vi "volume_viewer.vi"() -> ()   [LabVIEW 2024]
uses:
  <vilib>/sklein/WebView2/Webview2 Control/WebView2 Control.xctl
  definitions/local_volume.ctl
  definitions/local_issue.ctl
  definitions/comicvine_issue.generic_credit.ctl
  definitions/comicvine_issue.associated_image.ctl
  definitions/comicvine_issue.person_credit.ctl
  <vilib>/addons/_JKI Toolkits/State Machine/_JKI_lib_State_Machine.llb/Select State(s)_err__jki_lib_state_machine.vi
  <vilib>/addons/_JKI Toolkits/State Machine/_JKI_lib_State_Machine.llb/Periodic Trigger__ogtk__JKI-SM__jki_lib_state_machine.vi
  <userlib>/_OpenG.lib/file/file.llb/Strip Path Extension - String__ogtk.vi
  <userlib>/_OpenG.lib/file/file.llb/openg_file.lvlib
  <vilib>/addons/_JKI.lib/Serialization/JSON/JKI JSON Serialization.lvlib
panel:
  in  "issue detail tab control":enum32{"Details", "Cover", "Lists"}(tab)
  out "Issue ID":i32 caption="Numeric"
  out "Issue Title":string
  out "Cover Date":string
  out "Issue Number":string
  in  "issue description":string(xcontrol)
  in  "issue cover":string(xcontrol)
  out "Characters":string[](array[string])
  out "Teams":string[](array[string])
  out "StoryArcs":string[](array[string])
  out "Creators":string[](array[string])
  out "Concepts":string[](array[string])
  in  "sort volume":bool
  in  "to top":bool
  in  "move down":bool
  in  "move up":bool
  in  "issues":i32(listbox)
  out "Start Year":i32 caption="Numeric"
  out "Number of issues":i32 caption="Numeric"
  out "Sortable Title":string
  out "Title":string
  in  "volume description":string(xcontrol)
  in  "volumes":i32(listbox)
  in  "Folder":i32(listbox)
  in  "Exit":bool
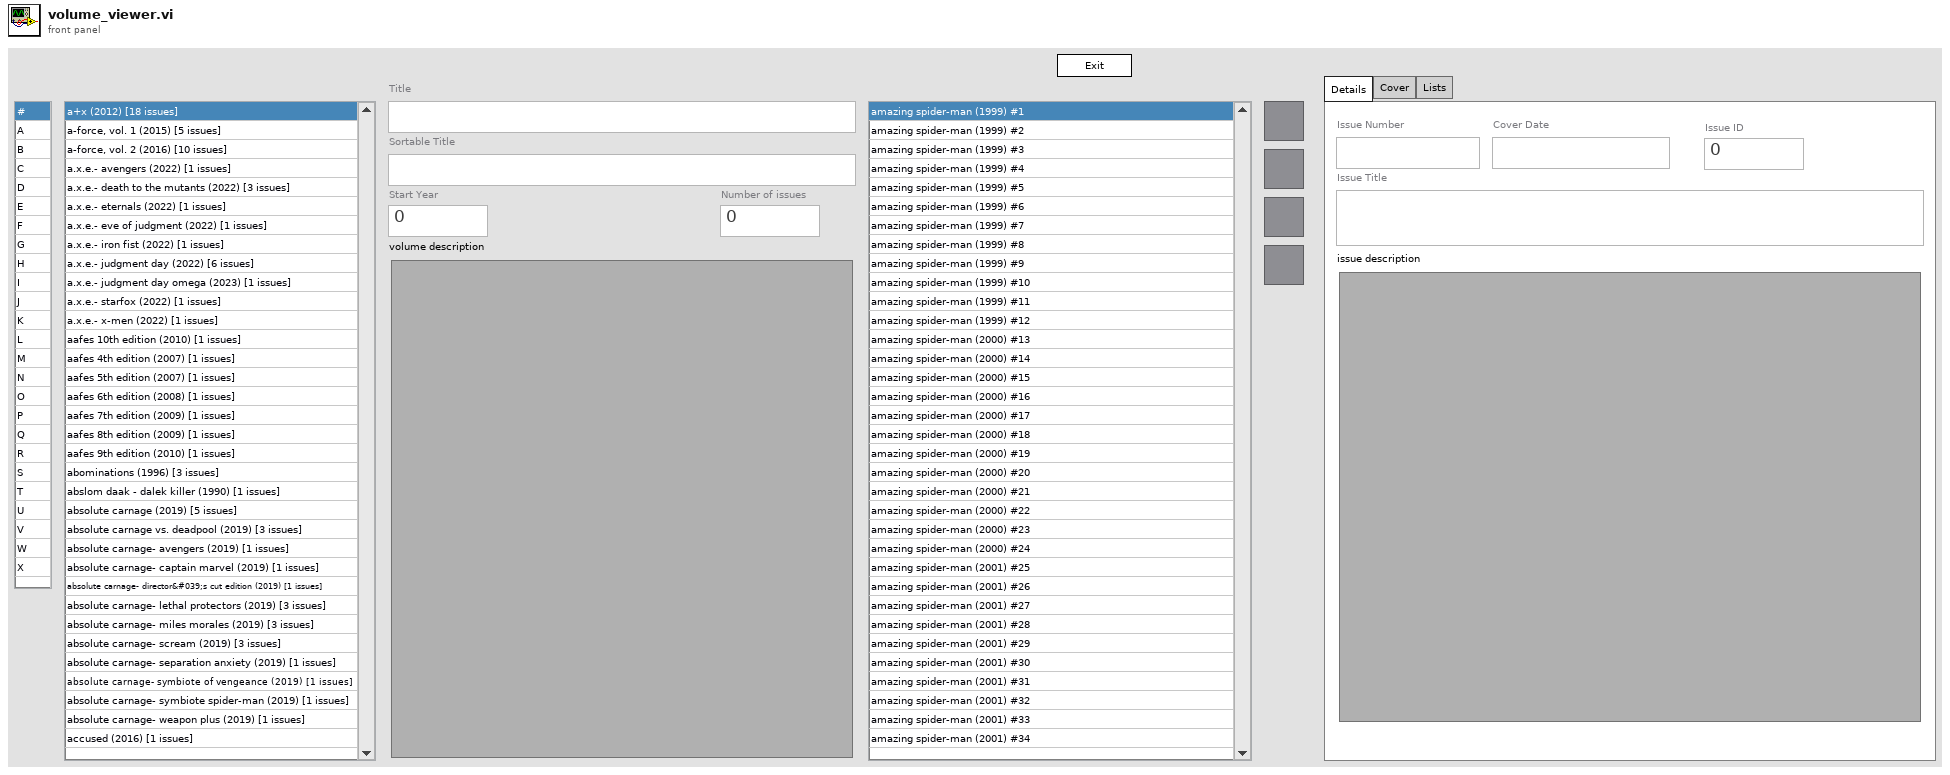
[diagram p1: front panel]
types:
  T1 = enum32{"Invalid", "Standard", "Closed", "Hidden", "Minimized", "Maximized"}
  T2 = enum32{"invalid app kind", "Development System", "Run Time System", "Student Edition", "Embedded LabVIEW", "Evaluation", "Custom"}
  T3 = typedef "local_volume.ctl" = cluster{"id":i32, "name":string, "name_sortable":string, "aliases":string[], "description":string, "url":string, "count_of_issues":i32, "start_year":i32, "publisher_id":i32, "issue_ids":i32[], "date_last_updated":timestamp, "volume":i32, "cv_id":string}
  T4 = typedef "local_issue.ctl" = cluster{"cover_date":timestamp, "id":i32, "cv_id":string, "name":string, "sortable_name":string, "issue_number":string, "deck":string, "description":string, "volume":T5, "store_date":timestamp, "date_last_updated":timestamp, "site_detail_url":string, "cover_url":string, "associated_images":T6[], "characters":T5[], "concepts":T5[], "creators":T7[], "storyArcs":T5[], "teams":T5[]}
  T5 = typedef "comicvine_issue.generic_credit.ctl" = cluster{"id":i32, "name":string}
  T6 = typedef "comicvine_issue.associated_image.ctl" = cluster{"original_url":string, "id":i32}
  T7 = typedef "comicvine_issue.person_credit.ctl" = cluster{"id":i32, "name":string, "role":string}
  T8 = cluster{"Core":cluster{"Current VI Reference":refnum<vi>, "Close Panel on Exit?":bool}, "cv_vols":path[], "vol_filter_map":map{i32, cluster{"name":string, "path":path}[]}, "current_vol_array":cluster{"name":string, "path":path}[], "volume":T3, "issues":T4[], "root paths":cluster{"cv_volumes":path, "cv_issues":path}}
  T9 = cluster{"Current VI Reference":refnum<vi>, "Close Panel on Exit?":bool}
  T10 = typedef "WebView2 Control.xctl/Events.ctl" = cluster{"Navigation Complete Event":refnum<user-event>, "Source Changed Event":refnum<user-event>, "Document Title Changed Event":refnum<user-event>, "Status Bar Text Changed":refnum<user-event>, "Web Message Received":refnum<user-event>, "Window Close Requested":refnum<user-event>, "DOM Loaded":refnum<user-event>, "Navigation Started Event":refnum<user-event>}
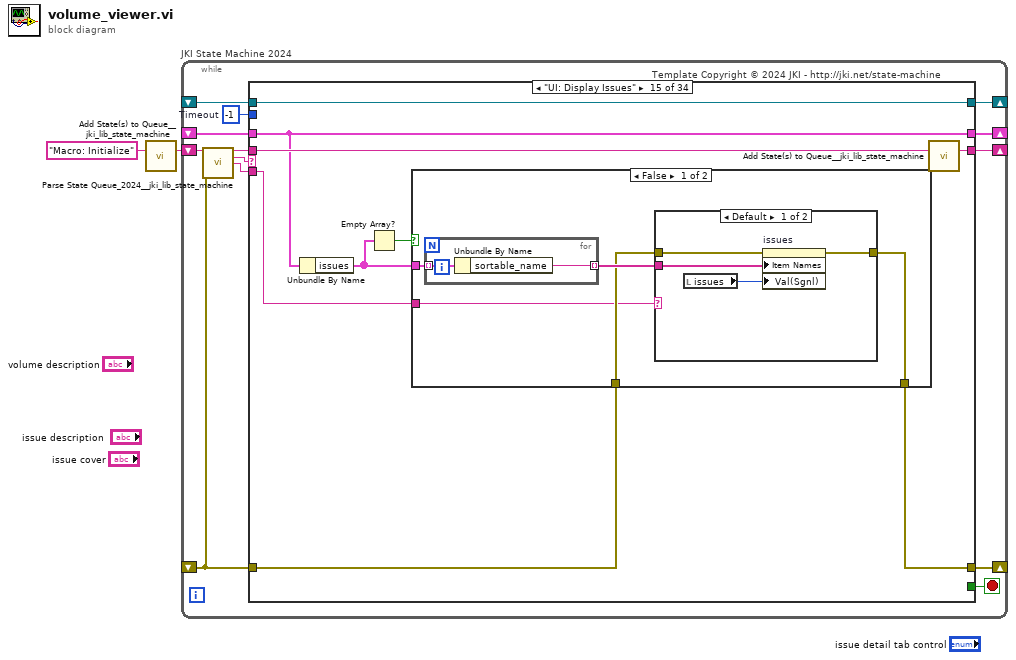
[diagram p0: block diagram]
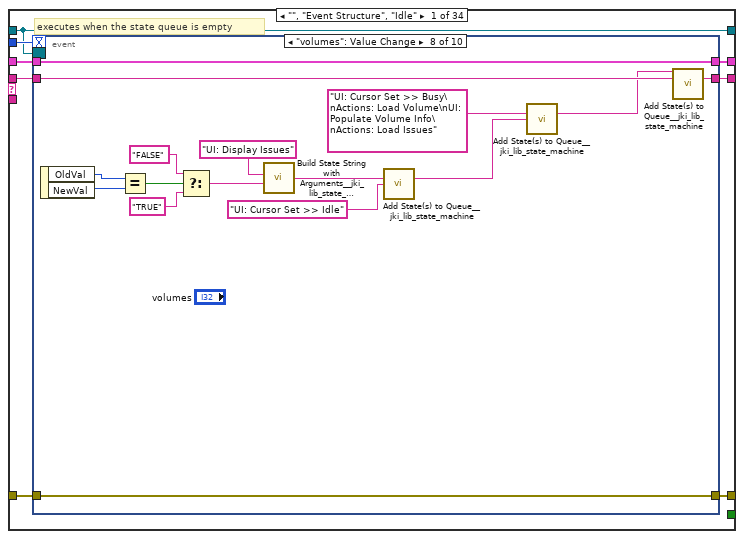
[diagram p2: hidden frame]
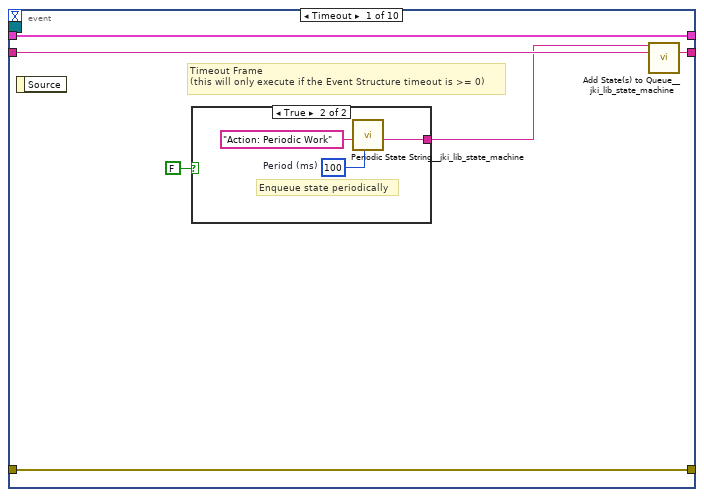
[diagram p3: hidden frame]
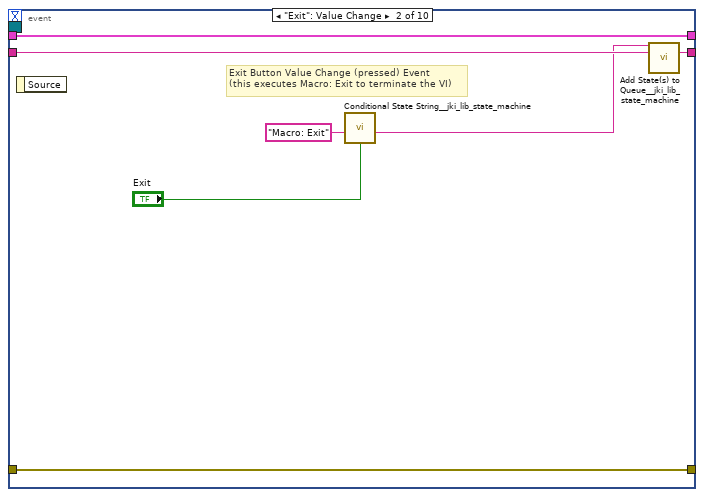
[diagram p5: hidden frame]
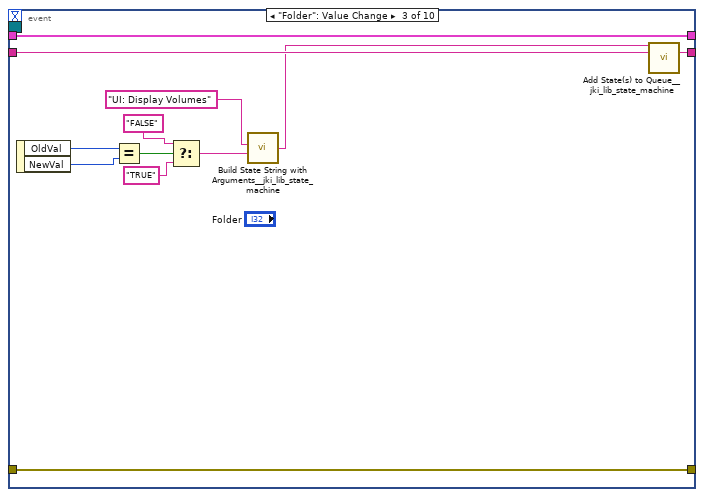
[diagram p6: hidden frame]
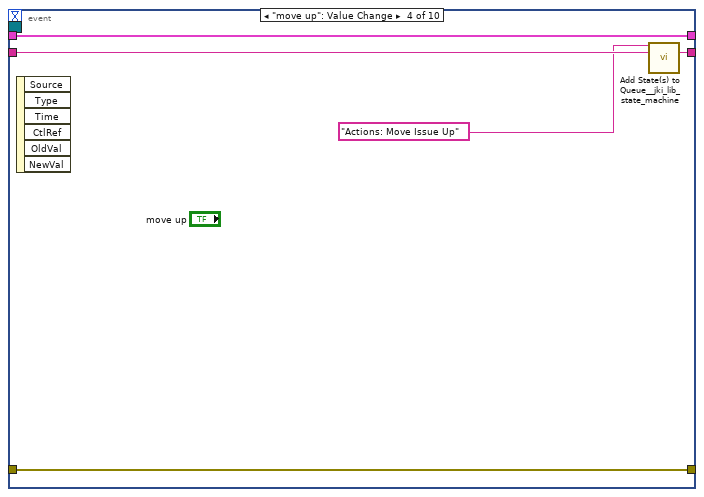
[diagram p7: hidden frame]
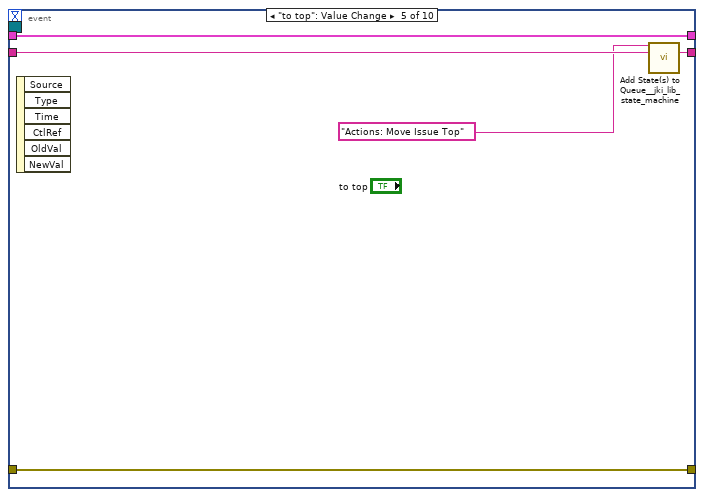
[diagram p8: hidden frame]
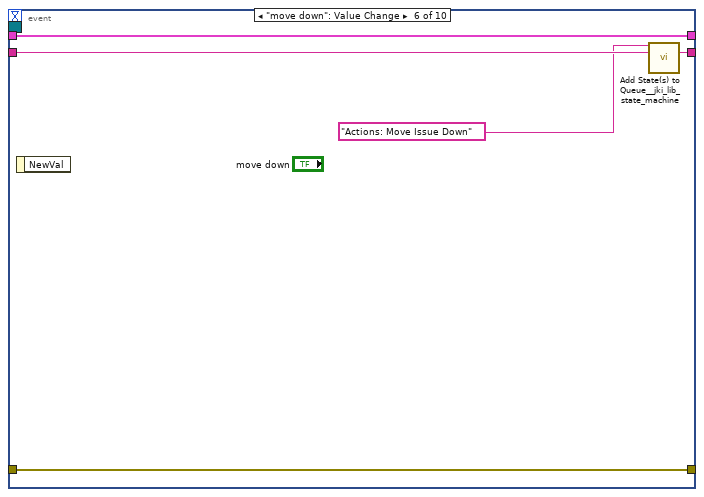
[diagram p9: hidden frame]
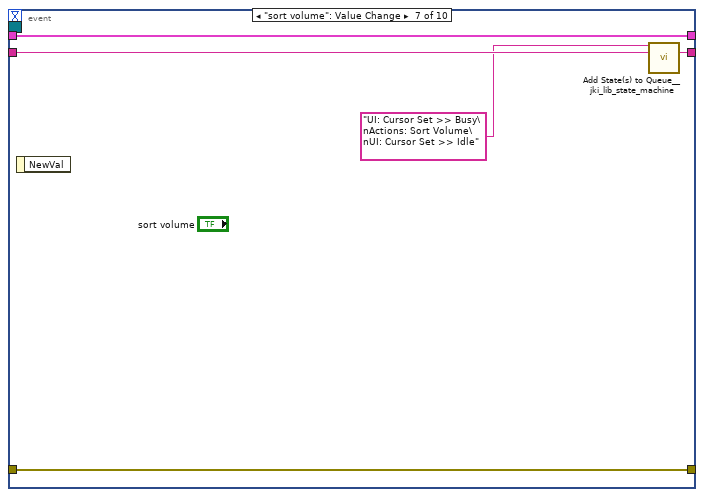
[diagram p10: hidden frame]
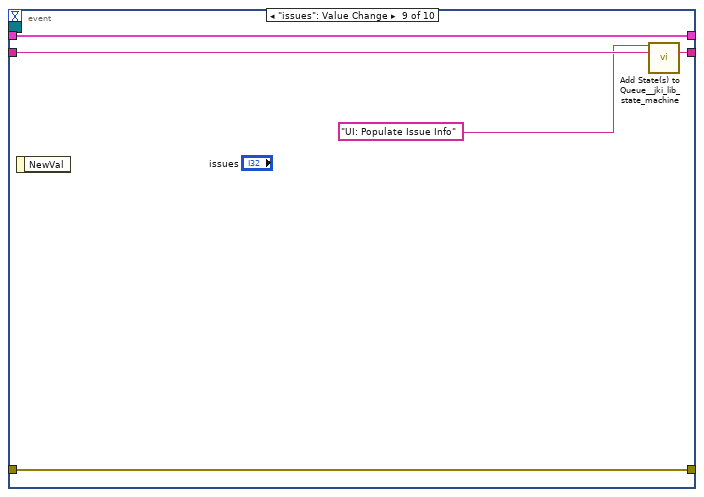
[diagram p11: hidden frame]
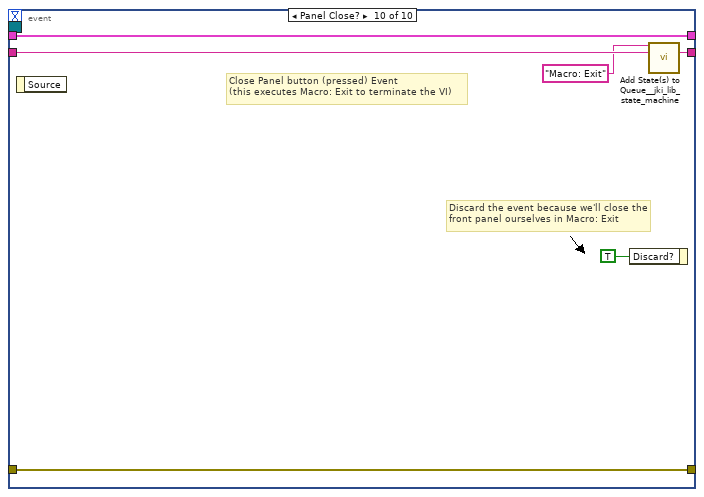
[diagram p12: hidden frame]
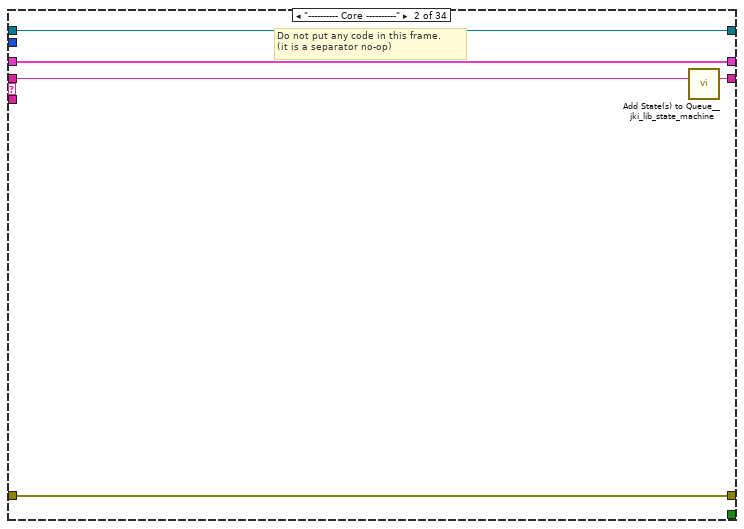
[diagram p13: hidden frame]
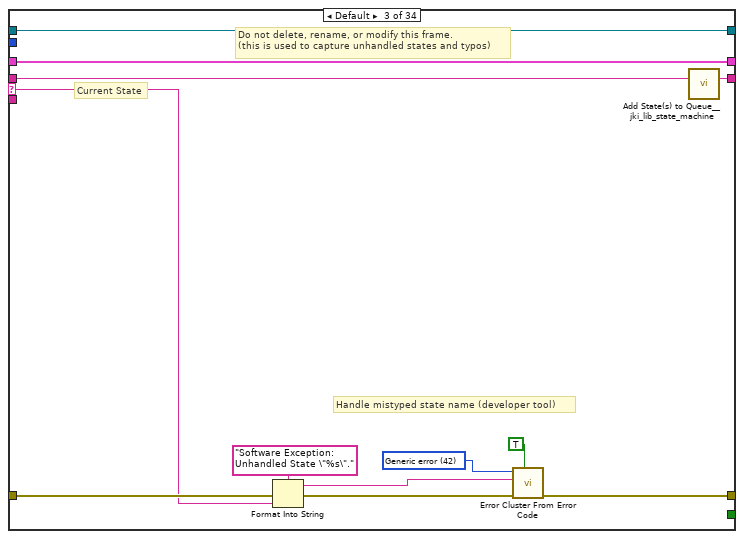
[diagram p14: hidden frame]
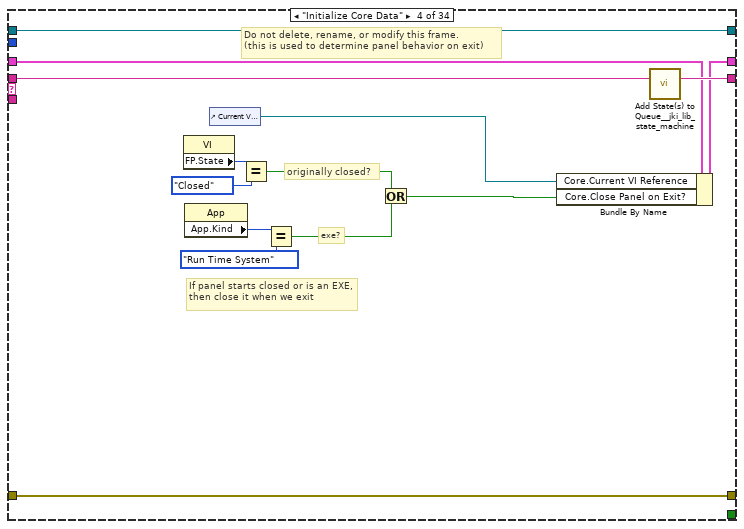
[diagram p15: hidden frame]
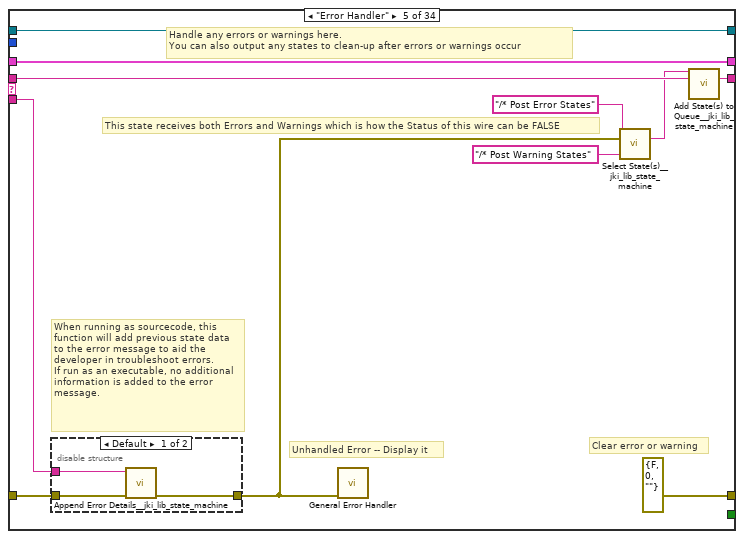
[diagram p16: hidden frame]
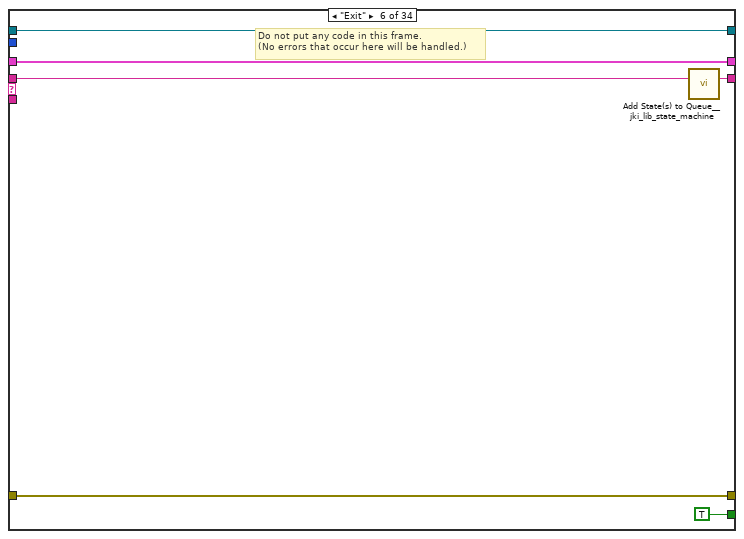
[diagram p18: hidden frame]
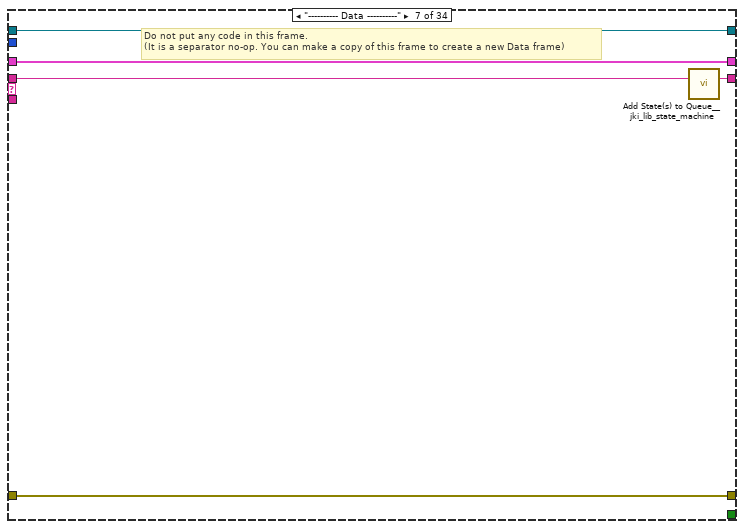
[diagram p19: hidden frame]
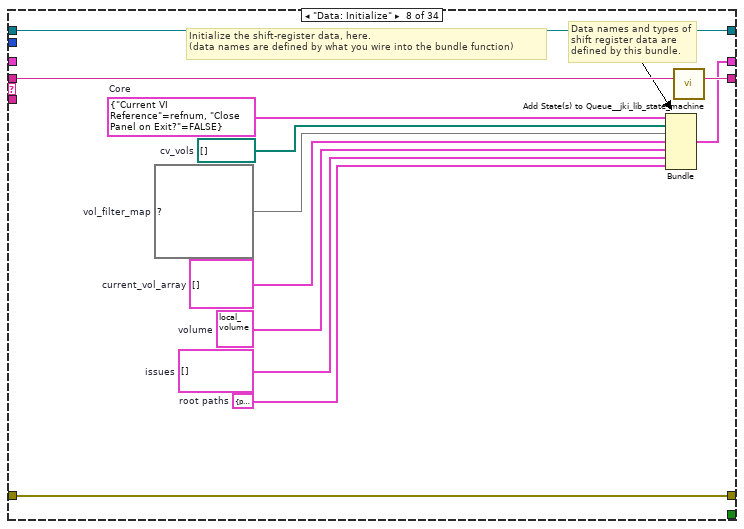
[diagram p20: hidden frame]
diagram:
  n1 = call <vilib>:"Add State(s) to Queue__jki_lib_state_machine.vi"("State(s) in (\"\")"="Macro: Initialize") -> ("States Out"=w2:string)  [unwired: 14 in]
  n2 = while "JKI State Machine 2024" {
    shift-right: [w8] -> _
    shift-left: _ -> [w7]
    shift-right: [w11] -> _
    shift-left: _ -> [w5]
    shift-right: [w10] -> _
    shift-left: w2 -> [w12]
    shift-right: [w4] -> _
    shift-left: _ -> [w3]
    stop <- w9 stop-if-true
    w6 = -1  # Timeout
    # "Template Copyright © 2024 JKI - http://jki.net/state-machine"
    n3 = call <vilib>:"Parse State Queue_2024__jki_lib_state_machine.vi"("State Queue"=w12, "Error In (no error)"=w5) -> ("Remaining States"=w14:string, "Current State"=w15:string, "Arguments"=w13:string)  [unwired: 11 in]
    n4 = case shown="\"UI: Display Issues\"" w15 {
      selector: w15 -> [_ _ w105 _ _ _ _ _ _ _ _ _ _ _ _ _ _ _ _ _ _ _ _ _ _ _ _ _ _ _ _ _ _ _]
      tunnel: w14 -> [w23 w103 w109 w129 w140 w150 w155 w167 w174 w179 w189 w195 w200 w213 w232 w253 w264 w294 w313 w318 w325 w337 w407 w413 w423 w428 w440 w462 w486 w508 w525 w536 w570 w581]
      tunnel: w13 -> [_ _ _ _ w135 _ _ _ _ _ _ _ _ w201 w224 _ _ _ _ _ w320 w331 _ _ _ _ _ _ _ _ _ _ _ _]
      tunnel: w7 -> [w21 w100 w107 w122 w137 w148 w152 _ w169 w176 w187 w193 w197 w209 w227 w250 w259 w291 w311 w316 w323 w333 w404 w410 w421 w425 w436 w459 w483 w505 w511 w530 w562 w576]
      tunnel: [w20 w101 w111 w126 errorcluster {"status"=FALSE, "code"=0, "source"=""} ("error out") w147 w153 w164 w170 w177 w181 w190 w198 w204 w228 w251 w261 w277 w310 w315 w321 w334 w405 w411 w418 w426 w432 w442 w465 w488 w513 w527 w565 w573] -> w11
      tunnel: w5 -> [w17 w101 w110 w126 w136 w147 w153 w164 w171 w177 w183 w191 w198 w205 w229 w251 w262 w280 w310 w315 w322 w335 w405 w411 w418 w426 w437 w449 w473 w495 w519 w531 w564 w572]
      tunnel: [w22 w102 w108 w128 w139 w149 w154 w166 w173 w178 w188 w194 w199 w212 w231 w252 w263 w293 w312 w317 w324 w336 w406 w412 w422 w427 w439 w461 w485 w507 w524 w535 w569 w581] -> w10
      tunnel: [_ _ _ _ _ TRUE _ _ _ _ _ _ _ _ _ _ _ _ _ _ _ _ _ _ _ _ _ _ _ _ _ _ _ _] -> w9
      tunnel: [w19 w100 w107 w127 w137 w148 w152 w165 w169 w176 w187 w193 w197 w208 w227 w250 w259 w291 w311 w316 w323 w333 w404 w410 w421 w425 w436 w459 w483 w505 w510 w528 w566 w574] -> w8
      tunnel: w6 -> [w18 _ _ _ _ _ _ _ _ _ _ _ _ _ _ _ _ _ _ _ _ _ _ _ _ _ _ _ _ _ _ _ _ _]
      tunnel: [w16 w99 w104 w116 w130 w145 w151 w159 w168 w175 w184 w192 w196 w203 w230 w249 w260 w292 w308 w314 w319 w330 w403 w408 w414 w424 w438 w460 w484 w506 w512 w534 w563 w571] -> w4
      tunnel: w3 -> [w16 w99 w104 w116 w130 w145 w151 w159 w168 w175 _ w192 w196 w203 w230 w249 w260 w292 w308 w314 w319 w330 w403 w408 w414 w424 w438 w460 w484 w506 w512 w534 w563 w571]
      frame "", "Event Structure", "Idle" {
        # "executes when the state queue is empty"
        n5 = event shown="[7] \"volumes\": Value Change" {
          selector: w16 -> [_ _ _ _ _ _ _ _ _ _]
          dyn-events: _ -> [_ _ _ _ _ _ _ _ _ _]
          timeout: w18 -> [_ _ _ _ _ _ _ _ _ _]
          tunnel: w23 -> [w29 w39 w51 w56 w61 w66 w71 w87 w92 w98]
          tunnel: [w28 w38 w50 w55 w60 w65 w70 w86 w91 w97] -> w22
          tunnel: w21 -> [w26 w36 w48 w53 w58 w63 w68 w84 w89 w95]
          tunnel: [w27 w37 w49 w54 w59 w64 w69 w85 w90 w96] -> w20
          tunnel: w17 -> [w27 w37 w49 w54 w59 w64 w69 w85 w90 w96]
          tunnel: [w26 w36 w48 w53 w58 w63 w68 w84 w89 w95] -> w19
          event Timeout {
            # "Timeout Frame\n(this will only execute if the Event Structure timeout is >= 0)"
            n6 = event-data() -> ()  [unwired: 1 in, 1 out]
            n7 = case shown="True" FALSE {
              tunnel: [_ w32] -> w25
              frame False {
              }
              frame True {
                w30 = u32 100  # Period (ms)
                # "Enqueue state periodically"
                n8 = call <vilib>:"Periodic State String__jki_lib_state_machine.vi"("Period (ms)"=w30, "State"="Action: Periodic Work") -> ("State Out"=w32:string)  [unwired: 9 in]
              }
            }
            n9 = call <vilib>:"Add State(s) to Queue__jki_lib_state_machine.vi"("State(s) in Front (\"\")"=w25, "State(s) in (\"\")"=w29) -> ("States Out"=w28:string)  [unwired: 13 in]
          }
          event "Exit": Value Change {
            # "Exit Button Value Change (pressed) Event\n(this executes Macro: Exit to terminate the VI)"
            n10 = event-data() -> ()  [unwired: 1 in, 1 out]
            n11 = call <vilib>:"Conditional State String__jki_lib_state_machine.vi"("Do State(s)?"="Exit", "State"="Macro: Exit") -> ("State Out"=w33:string)  [unwired: 7 in]
            n12 = call <vilib>:"Add State(s) to Queue__jki_lib_state_machine.vi"("State(s) in Front (\"\")"=w33, "State(s) in (\"\")"=w39) -> ("States Out"=w38:string)  [unwired: 13 in]
          }
          event "Folder": Value Change {
            n13 = event-data() -> ("OldVal"=w47:i32, "NewVal"=w46:i32)  [unwired: 1 in]
            n14 = Equal?(x=w47, y=w46) -> (x = y?=w45:bool)
            n15 = Select(t="FALSE", s=w45, f="TRUE") -> (s? t:f=w41:string)
            n16 = call <vilib>:"Build State String with Arguments__jki_lib_state_machine.vi"("Arguments (\"\")"=w41, "State"="UI: Display Volumes") -> ("State with Arguments"=w40:string)  [unwired: 4 in]
            n17 = call <vilib>:"Add State(s) to Queue__jki_lib_state_machine.vi"("State(s) in Front (\"\")"=w40, "State(s) in (\"\")"=w51) -> ("States Out"=w50:string)  [unwired: 13 in]
          }
          event "move up": Value Change {
            n18 = event-data() -> ()  [unwired: 1 in, 6 out]
            n19 = call <vilib>:"Add State(s) to Queue__jki_lib_state_machine.vi"("State(s) in Front (\"\")"="Actions: Move Issue Up", "State(s) in (\"\")"=w56) -> ("States Out"=w55:string)  [unwired: 13 in]
          }
          event "to top": Value Change {
            n20 = event-data() -> ()  [unwired: 1 in, 6 out]
            n21 = call <vilib>:"Add State(s) to Queue__jki_lib_state_machine.vi"("State(s) in Front (\"\")"="Actions: Move Issue Top", "State(s) in (\"\")"=w61) -> ("States Out"=w60:string)  [unwired: 13 in]
          }
          event "move down": Value Change {
            n22 = event-data() -> ()  [unwired: 1 in, 1 out]
            n23 = call <vilib>:"Add State(s) to Queue__jki_lib_state_machine.vi"("State(s) in Front (\"\")"="Actions: Move Issue Down", "State(s) in (\"\")"=w66) -> ("States Out"=w65:string)  [unwired: 13 in]
          }
          event "sort volume": Value Change {
            n24 = event-data() -> ()  [unwired: 1 in, 1 out]
            n25 = call <vilib>:"Add State(s) to Queue__jki_lib_state_machine.vi"("State(s) in Front (\"\")"="UI: Cursor Set >> Busy\nActions: Sort Volume\nUI: Cursor Set >> Idle", "State(s) in (\"\")"=w71) -> ("States Out"=w70:string)  [unwired: 13 in]
          }
          event "volumes": Value Change {
            n26 = event-data() -> ("OldVal"=w82:i32, "NewVal"=w83:i32)  [unwired: 1 in]
            n27 = Equal?(x=w82, y=w83) -> (x = y?=w79:bool)
            n28 = Select(t="FALSE", s=w79, f="TRUE") -> (s? t:f=w77:string)
            n29 = call <vilib>:"Build State String with Arguments__jki_lib_state_machine.vi"("Arguments (\"\")"=w77, "State"="UI: Display Issues") -> ("State with Arguments"=w74:string)  [unwired: 4 in]
            n30 = call <vilib>:"Add State(s) to Queue__jki_lib_state_machine.vi"("State(s) in (\"\")"=w74, "State(s) at Back (\"\")"="UI: Cursor Set >> Idle" ("State(s) at Back (\"\")")) -> ("States Out"=w73:string)  [unwired: 13 in]
            n31 = call <vilib>:"Add State(s) to Queue__jki_lib_state_machine.vi"("State(s) in (\"\")"="UI: Cursor Set >> Busy\nActions: Load Volume\nUI: Populate Volume Info\nActions: Load Issues", "State(s) at Back (\"\")"=w73) -> ("States Out"=w80:string)  [unwired: 13 in]
            n32 = call <vilib>:"Add State(s) to Queue__jki_lib_state_machine.vi"("State(s) in Front (\"\")"=w80, "State(s) in (\"\")"=w87) -> ("States Out"=w86:string)  [unwired: 13 in]
          }
          event "issues": Value Change {
            n33 = event-data() -> ()  [unwired: 1 in, 1 out]
            n34 = call <vilib>:"Add State(s) to Queue__jki_lib_state_machine.vi"("State(s) in Front (\"\")"="UI: Populate Issue Info", "State(s) in (\"\")"=w92) -> ("States Out"=w91:string)  [unwired: 13 in]
          }
          event Panel Close? {
            # "Discard the event because we'll close the front panel ourselves in Macro: Exit"
            # "Close Panel button (pressed) Event\n(this executes Macro: Exit to terminate the VI)"
            n35 = event-data() -> ()  [unwired: 1 in, 1 out]
            n36 = event-data("Discard?"=TRUE) -> ()  [unwired: 1 in, 1 out]
            n37 = call <vilib>:"Add State(s) to Queue__jki_lib_state_machine.vi"("State(s) in Front (\"\")"="Macro: Exit", "State(s) in (\"\")"=w98) -> ("States Out"=w97:string)  [unwired: 13 in]
          }
        }
      }
      frame "---------- Core ----------" {
        # "Do not put any code in this frame.\n(it is a separator no-op)"
        n38 = call <vilib>:"Add State(s) to Queue__jki_lib_state_machine.vi"("State(s) in (\"\")"=w103) -> ("States Out"=w102:string)  [unwired: 14 in]
      }
      frame Default {
        w114 = 42 items=["No error", "Argument error", "Memory is full", "Out of zone", "End of file", "File already open", "Generic file I/O error", "File not found", "File permission error", "Disk is full", "Duplicate path", "Too many files open", "System feature not enabled", "Resource file not found", "Cannot add resource", "Resource not found", "Image not found", "Image memory error", "Pen does not exist", "Config type invalid", "Config token not found", "Config parse error", "Config memory error", "Bad external code format", "Bad external code offset", "External code not present", "Null window", "Destroy window error", "Null menu", "Print aborted", "Bad print record", "Print driver error", "Windows error during printing", "Memory error during printing", "Print dialog error", "Generic print error", "Invalid device refnum", "Device not found", "Device parameter error", "Device unit error", "Cannot open device", "Device call aborted", "Generic error", "Cancelled by user", "Object ID too low", "Object ID too high", "Object not in heap", "Unknown heap", "Unknown object (invalid DefProc)", "Unknown object (DefProc not in table)", "Message out of range", "Invalid (null) method", "Unknown message", "Manager call not supported", "Bad address", "Network operation in progress", "Network operation timed out", "Connection is busy", "Network attribute not supported", "Network error", "Address in use", "System out of memory", "Connection aborted", "Connection refused", "Not connected", "Already connected", "Connection closed", "Initialization error (interapplication manager)", "Bad occurrence", "Wait on unbound occurrence handler", "Occurrence queue overflow", "Datalog type conflict", "Unused", "Unrecognized type (interapplication manager)", "Memory corrupt", "Failed to make temporary DLL", "Old CIN version", "Drag socket not found", "Failed to load drop-object", "Failed to register OLE object", "Failed to release OLE object", "Format specifier type mismatch", "Unknown format specifier", "Too few format specifiers", "Too many format specifiers", "Scan failed", "Newer CIN version", "Error converting to variant", "Runtime menu error", "Password tampered", "Variant attribute not found", "Incompatible variant data type", "Event data is not available", "Event Store is not present", "Occurrence is not found", "Event Queue is not created", "Event info is not available", "Refnum passed is NULL", "Error retrieving Class GUID", "Error retrieving CoClass GUID", "Error retrieving TypeLib GUID.", "Bad built application magic bytes.", "Specific driver is different from the specific driver associated with the Logical Name.", "There is no session opened to the class driver.", "Max Error", "MAX - Error with config objects", "MAX - Error loading configuration", "MAX - Group not supported"]
        # "Current State"
        # "Do not delete, rename, or modify this frame.\n(this is used to capture unhandled states and typos)"
        # "Handle mistyped state name (developer tool)"
        n39 = Format Into String(format string="Software Exception: Unhandled State \"%s\"." ("message"), error in=w110, w105) -> (resulting string=w113:string, error out=w112:errorcluster)  [unwired: 1 in]
        n40 = call <vilib>:"Error Cluster From Error Code.vi"("show call chain? (False)"=TRUE, "error in (no error)"=w112, "error message (\"\")"=w113, "error code (0)"=w114) -> ("error out"=w111:errorcluster)  [unwired: 5 in]
        n41 = call <vilib>:"Add State(s) to Queue__jki_lib_state_machine.vi"("State(s) in (\"\")"=w109) -> ("States Out"=w108:string)  [unwired: 14 in]
      }
      frame "Initialize Core Data" {
        # "Do not delete, rename, or modify this frame.\n(this is used to determine panel behavior on exit)"
        # "originally closed?"
        # "exe?"
        # "If panel starts closed or is an EXE, then close it when we exit"
        n42 = property class="VI"() -> ("FP.State"=w119:T1)  [unwired: 2 in, 2 out]
        n43 = property class="App"() -> ("App.Kind"=w125:T2)  [unwired: 2 in, 2 out]
        n44 = control-ref of="Current VI Reference"() -> (w120:refnum<vi>)
        n45 = Equal?(x=w119, y=T1."Closed" ("Front Panel Window:State")) -> (x = y?=w117:bool)
        n46 = Equal?(x=w125, y=T2."Run Time System" ("Application:Kind")) -> (x = y?=w123:bool)
        n47 = Or(x=w117, y=w123) -> (x .or. y?=w121:bool)
        n48 = Bundle By Name(cluster=w122, "Core.Current VI Reference"=w120, "Core.Close Panel on Exit?"=w121) -> (w127:T8)
        n49 = call <vilib>:"Add State(s) to Queue__jki_lib_state_machine.vi"("State(s) in (\"\")"=w129) -> ("States Out"=w128:string)  [unwired: 14 in]
      }
      frame "Error Handler" {
        # "When running as sourcecode, this function will add previous state data to the error message to aid the developer in troubleshoot errors.\nIf run as an executable, no additional information is added to the error message."
        # "This state receives both Errors and Warnings which is how the Status of this wire can be FALSE"
        # "Unhandled Error -- Display it"
        # "Handle any errors or warnings here.\nYou can also output any states to clean-up after errors or warnings occur"
        # "Clear error or warning"
        n50 = disable-structure shown="Default" {
          disable-tunnel: w136 -> [w143 w144]
          disable-tunnel: w135 -> [w142 _]
          disable-tunnel: [w141 w144] -> w134
          frame condition #0 (active) {
            n51 = call <vilib>:"Append Error Details__jki_lib_state_machine.vi"("error in (no error)"=w143, "Previous State and Argument(s)"=w142) -> ("error out"=w141:errorcluster)  [unwired: 9 in]
          }
          frame condition #1 {
          }
        }
        n52 = call <vilib>:"General Error Handler.vi"("error in (no error)"=w134) -> ()  [unwired: 10 in, 5 out]
        n53 = call-poly <vilib>:"Select State(s)__jki_lib_state_machine.vi"("State(s) if True (\"\")"="/* Post Error States", "Select"=w134, "State(s) if False (\"\")"="/* Post Warning States") -> ("States Out"=w132:string)  [unwired: 12 in]
        n54 = call <vilib>:"Add State(s) to Queue__jki_lib_state_machine.vi"("State(s) in Front (\"\")"=w132, "State(s) in (\"\")"=w140) -> ("States Out"=w139:string)  [unwired: 13 in]
      }
      frame "Exit" {
        # "Do not put any code in this frame.\n(No errors that occur here will be handled.)"
        n55 = call <vilib>:"Add State(s) to Queue__jki_lib_state_machine.vi"("State(s) in (\"\")"=w150) -> ("States Out"=w149:string)  [unwired: 14 in]
      }
      frame "---------- Data ----------" {
        # "Do not put any code in this frame.\n(It is a separator no-op. You can make a copy of this frame to create a new Data frame)"
        n56 = call <vilib>:"Add State(s) to Queue__jki_lib_state_machine.vi"("State(s) in (\"\")"=w155) -> ("States Out"=w154:string)  [unwired: 14 in]
      }
      frame "Data: Initialize" {
        w156 = cluster{"cv_volumes":path, "cv_issues":path} {"cv_volumes"=path "D:/Comics/data/cv_volumes", "cv_issues"=path "D:/Comics/data/cv_issues"}  # root paths
        w157 = T4[] []  # issues
        w158 = T3 {"id"=0, "name"="", "name_sortable"="", "aliases"=[], "description"="", "url"="", "count_of_issues"=0, "start_year"=0, "publisher_id"=0, "issue_ids"=[], "date_last_updated"=timestamp(0 s since 1904-01-01), "volume"=0, "cv_id"=""}  # volume
        w160 = cluster{"name":string, "path":path}[] []  # current_vol_array
        w161 = map{i32, cluster{"name":string, "path":path}[]} {}  # vol_filter_map
        w162 = path[] []  # cv_vols
        w163 = T9 {"Current VI Reference"=refnum, "Close Panel on Exit?"=FALSE}  # Core
        # "Data names and types of shift register data are defined by this bundle."
        # "Initialize the shift-register data, here.\n(data names are defined by what you wire into the bundle function)"
        n57 = Bundle("Core"=w163, "cv_vols"=w162, "vol_filter_map"=w161, "current_vol_array"=w160, "volume"=w158, "issues"=w157, "root paths"=w156) -> (w165:T8)  [unwired: 1 in]
        n58 = call <vilib>:"Add State(s) to Queue__jki_lib_state_machine.vi"("State(s) in (\"\")"=w167) -> ("States Out"=w166:string)  [unwired: 14 in]
      }
      frame "Data: Cleanup" {
        # "Cleanup any data and references, here.\n(this is called automatically, by the Macro: Exit)"
        n59 = Unbundle By Name(w169) -> ("Core.Current VI Reference"=w172:refnum<vi>)
        n60 = Close Reference(reference=w172, error in (no error)=w171) -> (error out=w170:errorcluster)
        n61 = call <vilib>:"Add State(s) to Queue__jki_lib_state_machine.vi"("State(s) in (\"\")"=w174) -> ("States Out"=w173:string)  [unwired: 14 in]
      }
      frame "---------- Events ----------" {
        n62 = call <vilib>:"Add State(s) to Queue__jki_lib_state_machine.vi"("State(s) in (\"\")"=w179) -> ("States Out"=w178:string)  [unwired: 14 in]
      }
      frame "Events: Register" {
        w185 = cluster{"My Event Data":bool} {"My Event Data"=FALSE}  # My User Event
        n63 = Create User Event(user event datatype=w185, error in=w183) -> (user event=w186:refnum<user-event>, error out=w182:errorcluster)
        n64 = property on="volume description" class="WebView2 Control (strict)"() -> ("Events"=w180:T10)  [unwired: 2 in, 2 out]
        n65 = register-events(error in=w182, w186, w180) -> (reference out=w184:refnum<event-registration>, error out=w181:errorcluster)  [unwired: 1 in]
        n66 = call <vilib>:"Add State(s) to Queue__jki_lib_state_machine.vi"("State(s) in (\"\")"=w189) -> ("States Out"=w188:string)  [unwired: 14 in]
      }
      frame "Events: Unregister" {
        n67 = Unregister For Events(event registration refnum=w192, error in=w191) -> (error out=w190:errorcluster)
        n68 = call <vilib>:"Add State(s) to Queue__jki_lib_state_machine.vi"("State(s) in (\"\")"=w195) -> ("States Out"=w194:string)  [unwired: 14 in]
      }
      frame "---------- UI ----------" {
        n69 = call <vilib>:"Add State(s) to Queue__jki_lib_state_machine.vi"("State(s) in (\"\")"=w200) -> ("States Out"=w199:string)  [unwired: 14 in]
      }
      frame "UI: Display Volumes" {
        n70 = Unbundle By Name(w209) -> ("vol_filter_map"=w211:map{i32, cluster{"name":string, "path":path}[]})
        n71 = local read "Folder"() -> (w210:i32)
        n72 = Look In Map(map=w211, key=w210) -> (value=w207:cluster{"name":string, "path":path}[])  [unwired: 1 in, 1 out]
        n73 = for {
          tunnel: w207 -> [w223] mode=indexing
          tunnel: [w222] -> w206 mode=indexing
          n74 = Unbundle By Name(w223) -> ("name"=w222:string)
        }
        n75 = local read "volumes"() -> (w202:i32)
        n76 = Bundle By Name(cluster=w209, "current_vol_array"=w207) -> (w208:T8)
        n77 = case shown="Default" w201 {
          tunnel: w206 -> [w217 w221]
          tunnel: w205 -> [w216 w220]
          tunnel: [w215 w219] -> w204
          tunnel: w202 -> [_ w218]
          frame "TRUE" {
            w214 = 0 ("Value (Signaling)")
            n78 = property on="volumes" class="LstBox (strict)"(error in=w216, "Item Names"=w217, "Val(Sgnl)"=w214, "Top Row"=w214) -> (error out=w215:errorcluster)  [unwired: 1 in, 1 out]
          }
          frame Default {
            n79 = property on="volumes" class="LstBox (strict)"(error in=w220, "Item Names"=w221, "Val(Sgnl)"=w218) -> (error out=w219:errorcluster)  [unwired: 1 in, 1 out]
          }
        }
        n80 = call <vilib>:"Add State(s) to Queue__jki_lib_state_machine.vi"("State(s) in (\"\")"=w213) -> ("States Out"=w212:string)  [unwired: 14 in]
      }
      frame "UI: Display Issues" {
        n81 = Unbundle By Name(w227) -> ("issues"=w226:T4[])
        n82 = Empty Array?(array=w226) -> (empty?=w225:bool)
        n83 = case shown="False" w225 {
          tunnel: w229 -> [w236 w248]
          tunnel: [w235 w248] -> w228
          tunnel: w226 -> [w234 _]
          tunnel: w224 -> [w233 _]
          frame False {
            n84 = for {
              tunnel: w234 -> [w247] mode=indexing
              tunnel: [w246] -> w237 mode=indexing
              n85 = Unbundle By Name(w247) -> ("sortable_name"=w246:string)
            }
            n86 = case shown="Default" w233 {
              tunnel: w237 -> [w241 w245]
              tunnel: w236 -> [w240 w244]
              tunnel: [w239 w243] -> w235
              frame Default {
                n87 = local read "issues"() -> (w238:i32)
                n88 = property on="issues" class="LstBox (strict)"(error in=w240, "Item Names"=w241, "Val(Sgnl)"=w238) -> (error out=w239:errorcluster)  [unwired: 1 in, 1 out]
              }
              frame "TRUE" {
                w242 = 0 ("Value (Signaling)")
                n89 = property on="issues" class="LstBox (strict)"(error in=w244, "Item Names"=w245, "Val(Sgnl)"=w242, "Top Row"=w242) -> (error out=w243:errorcluster)  [unwired: 1 in, 1 out]
              }
            }
          }
          frame True {
          }
        }
        n90 = call <vilib>:"Add State(s) to Queue__jki_lib_state_machine.vi"("State(s) in (\"\")"=w232) -> ("States Out"=w231:string)  [unwired: 14 in]
      }
      frame "UI: Ready" {
        n91 = call <vilib>:"Add State(s) to Queue__jki_lib_state_machine.vi"("State(s) in (\"\")"=w253) -> ("States Out"=w252:string)  [unwired: 14 in]
      }
      frame "UI: Populate Volume Info" {
        n92 = Unbundle By Name(w259) -> ("volume.start_year"=→"Start Year":i32, "volume.count_of_issues"=→"Number of issues":i32, "volume.name_sortable"=→"Sortable Title":string, "volume.name"=→"Title":string, "volume.description"=w254:string)
        n93 = property on="volume description" class="WebView2 Control (strict)"(error in=w262, "Document Source"=w254) -> (error out=w261:errorcluster)  [unwired: 1 in, 1 out]
        n94 = call <vilib>:"Add State(s) to Queue__jki_lib_state_machine.vi"("State(s) in (\"\")"=w264) -> ("States Out"=w263:string)  [unwired: 14 in]
      }
      frame "UI: Populate Issue Info" {
        n95 = Unbundle By Name(w291) -> ("issues"=w290:T4[])
        n96 = local read "issues"() -> (w289:i32)
        n97 = Index Array(array=w290, index=w289) -> (element=w288:T4)
        n98 = Unbundle By Name(w288) -> ("cover_date"=w287:timestamp, "id"=→"Issue ID":i32, "name"=→"Issue Title":string, "issue_number"=→"Issue Number":string, "cover_url"=w281:string, "description"=w276:string, "characters"=w275:T5[], "concepts"=w273:T5[], "storyArcs"=w271:T5[], "teams"=w269:T5[], "creators"=w267:T7[])
        n99 = property on="issue description" class="WebView2 Control (strict)"(error in=w280, "Document Source"=w276) -> (error out=w279:errorcluster)  [unwired: 1 in, 1 out]
        n100 = Format Date/Time String(time format string (%c)="%B %d, %Y", seconds (now)=w287) -> (date/time string=→"Cover Date":string)  [unwired: 1 in]
        n101 = property on="issue cover" class="WebView2 Control (strict)"(error in=w280, "URL"=w281) -> (error out=w278:errorcluster)  [unwired: 1 in, 1 out]
        n102 = for {
          tunnel: w275 -> [w307] mode=indexing
          tunnel: [w306] -> w274 mode=indexing
          n103 = Unbundle By Name(w307) -> ("name"=w306:string)
        }
        "Characters" <- w274
        n104 = for {
          tunnel: w273 -> [w305] mode=indexing
          tunnel: [w304] -> w272 mode=indexing
          n105 = Unbundle By Name(w305) -> ("name"=w304:string)
        }
        "Concepts" <- w272
        n106 = for {
          tunnel: w271 -> [w303] mode=indexing
          tunnel: [w302] -> w270 mode=indexing
          n107 = Unbundle By Name(w303) -> ("name"=w302:string)
        }
        "StoryArcs" <- w270
        n108 = for {
          tunnel: w269 -> [w301] mode=indexing
          tunnel: [w300] -> w268 mode=indexing
          n109 = Unbundle By Name(w301) -> ("name"=w300:string)
        }
        "Teams" <- w268
        n110 = Merge Errors(w278, w279) -> (w277:errorcluster)
        n111 = for {
          tunnel: w267 -> [w299] mode=indexing
          tunnel: [w296] -> w266 mode=indexing
          tunnel: " - " ("string") -> [w295]
          n112 = Unbundle By Name(w299) -> ("name"=w298:string, "role"=w297:string)
          n113 = Concatenate Strings(w298, w295, w297) -> (w296:string)
        }
        "Creators" <- w266
        n114 = call <vilib>:"Add State(s) to Queue__jki_lib_state_machine.vi"("State(s) in (\"\")"=w294) -> ("States Out"=w293:string)  [unwired: 14 in]
      }
      frame "UI: Initialize" {
        # "Initialize the User Interface, here.\n(this is called automatically, by the Macro: Initialize)"
        n115 = call <vilib>:"Add State(s) to Queue__jki_lib_state_machine.vi"("State(s) in Front (\"\")"="Actions: Populate cv_vols\nActions: create volume filter map\nUI: Display Volumes >> TRUE\nActions: Load Volume\nUI: Ready" ("State(s) in Front (\"\")"), "State(s) in (\"\")"=w313) -> ("States Out"=w312:string)  [unwired: 13 in]
      }
      frame "UI: Uninitialize" {
        # "Cleanup the User Interface, here.\n(this is called automatically, by the Macro: Exit)"
        n116 = call <vilib>:"Add State(s) to Queue__jki_lib_state_machine.vi"("State(s) in (\"\")"=w318) -> ("States Out"=w317:string)  [unwired: 14 in]
      }
      frame "UI: Cursor Set" {
        # "Argument"
        # "Set and Unset Cursor Busy.\n(Usage: \"UI: Cursor Set >> Busy|Idle\")"
        n117 = case shown="\"Idle\", Default" w320 {
          tunnel: w322 -> [w327 w329]
          tunnel: [w326 w328] -> w321
          frame "Idle", Default {
            n118 = call <vilib>:"Unset Busy.vi"("error in (no error)"=w327) -> ("error out"=w326:errorcluster)  [unwired: 10 in]
          }
          frame "Busy" {
            n119 = call <vilib>:"Set Busy.vi"("error in (no error)"=w329) -> ("error out"=w328:errorcluster)  [unwired: 9 in, 1 out]
          }
        }
        n120 = call <vilib>:"Add State(s) to Queue__jki_lib_state_machine.vi"("State(s) in (\"\")"=w325) -> ("States Out"=w324:string)  [unwired: 14 in]
      }
      frame "UI: Front Panel State" {
        # "Argument"
        # "Set Front Panel Open or Closed\n(Usage: \"UI: Front Panel State >> Open|Close\")"
        n121 = Unbundle By Name(w333) -> ("Core.Current VI Reference"=w332:refnum<vi>)
        n122 = case shown="\"Open\", \"Standard\", Default" w331 {
          tunnel: w335 -> [w343 w358 w369 w382 w395]
          tunnel: [w345 w359 w371 w384 w397] -> w334
          tunnel: w332 -> [w344 w356 w370 w383 w396]
          frame "Open", "Standard", Default {
            w338 = T1."Standard" ("State")
            n123 = property class="VI"(reference=w344, error in=w343) -> (reference out=w341:refnum<vi>, error out=w342:errorcluster, "FP.State"=w340:T1)
            n124 = Not Equal?(x=w340, y=w338) -> (x != y?=w339:bool)
            n125 = case shown="False" w339 {
              tunnel: [w349 w351] -> w345
              tunnel: w342 -> [w348 w351]
              tunnel: w341 -> [w347 _]
              tunnel: w338 -> [w346 _]
              frame True {
                n126 = invoke class="VI" method="FP.Open"(reference=w347, error in=w348, "Activate"=TRUE, "State"=w346) -> (error out=w349:errorcluster)  [unwired: 1 in, 4 out]
              }
              frame False {
              }
            }
          }
          frame "Close", "Closed" {
            n127 = property class="VI"(reference=w356, error in=w358) -> (reference out=w355:refnum<vi>, error out=w357:errorcluster, "FP.State"=w353:T1)
            n128 = Not Equal?(x=w353, y=T1."Closed" ("Front Panel Window:State")) -> (x != y?=w352:bool)
            n129 = case shown="True" w352 {
              tunnel: [w360 w363] -> w359
              tunnel: w357 -> [w360 w362]
              tunnel: w355 -> [_ w361]
              frame False {
              }
              frame True {
                n130 = invoke class="VI" method="FP.Close"(reference=w361, error in=w362) -> (error out=w363:errorcluster)  [unwired: 1 in, 2 out]
              }
            }
          }
          frame "Hidden", "Hide" {
            w364 = T1."Hidden" ("State")
            n131 = property class="VI"(reference=w370, error in=w369) -> (reference out=w367:refnum<vi>, error out=w368:errorcluster, "FP.State"=w366:T1)
            n132 = Not Equal?(x=w366, y=w364) -> (x != y?=w365:bool)
            n133 = case shown="True" w365 {
              tunnel: [w375 w376] -> w371
              tunnel: w368 -> [w374 w376]
              tunnel: w367 -> [w373 _]
              tunnel: w364 -> [w372 _]
              frame True {
                n134 = invoke class="VI" method="FP.Open"(reference=w373, error in=w374, "State"=w372) -> (error out=w375:errorcluster)  [unwired: 2 in, 4 out]
              }
              frame False {
              }
            }
          }
          frame "Minimize", "Minimized" {
            w377 = T1."Minimized" ("State")
            n135 = property class="VI"(reference=w383, error in=w382) -> (reference out=w380:refnum<vi>, error out=w381:errorcluster, "FP.State"=w379:T1)
            n136 = Not Equal?(x=w379, y=w377) -> (x != y?=w378:bool)
            n137 = case shown="True" w378 {
              tunnel: [w388 w389] -> w384
              tunnel: w381 -> [w387 w389]
              tunnel: w380 -> [w386 _]
              tunnel: w377 -> [w385 _]
              frame True {
                n138 = invoke class="VI" method="FP.Open"(reference=w386, error in=w387, "State"=w385) -> (error out=w388:errorcluster)  [unwired: 2 in, 4 out]
              }
              frame False {
              }
            }
          }
          frame "Maximize", "Maximized" {
            w390 = T1."Maximized" ("State")
            n139 = property class="VI"(reference=w396, error in=w395) -> (reference out=w393:refnum<vi>, error out=w394:errorcluster, "FP.State"=w392:T1)
            n140 = Not Equal?(x=w392, y=w390) -> (x != y?=w391:bool)
            n141 = case shown="True" w391 {
              tunnel: [w401 w402] -> w397
              tunnel: w394 -> [w400 w402]
              tunnel: w393 -> [w399 _]
              tunnel: w390 -> [w398 _]
              frame True {
                n142 = invoke class="VI" method="FP.Open"(reference=w399, error in=w400, "State"=w398) -> (error out=w401:errorcluster)  [unwired: 2 in, 4 out]
              }
              frame False {
              }
            }
          }
        }
        n143 = call <vilib>:"Add State(s) to Queue__jki_lib_state_machine.vi"("State(s) in (\"\")"=w337) -> ("States Out"=w336:string)  [unwired: 14 in]
      }
      frame "---------- Macro ----------" {
        # "Do not put any code in this frame.\n(It is a separator no-op. You can make a copy of this frame to create a new Macro frame)"
        n144 = call <vilib>:"Add State(s) to Queue__jki_lib_state_machine.vi"("State(s) in (\"\")"=w407) -> ("States Out"=w406:string)  [unwired: 14 in]
      }
      frame "Macro: Initialize" {
        # "Initialization Macro\n(This is called once, when the VI starts)"
        n145 = call <vilib>:"Add State(s) to Queue__jki_lib_state_machine.vi"("State(s) in Front (\"\")"="Data: Initialize\nInitialize Core Data\nEvents: Register\nUI: Initialize\nUI: Front Panel State >> Open", "State(s) in (\"\")"=w413) -> ("States Out"=w412:string)  [unwired: 13 in]
      }
      frame "Macro: Exit" {
        # "Exit Macro\n(This is called once, when the VI exits)"
        n146 = Unbundle By Name(w421) -> ("Core.Close Panel on Exit?"=w416:bool)
        n147 = call <vilib>:"Conditional State String__jki_lib_state_machine.vi"("Do State(s)?"=w416, "State"="UI: Front Panel State >> Close") -> ("State Out"=w415:string)  [unwired: 7 in]
        n148 = call <vilib>:"Add State(s) to Queue__jki_lib_state_machine.vi"("State(s) in (\"\")"=w415, "State(s) at Back (\"\")"="UI: Uninitialize\nData: Cleanup\nEvents: Unregister\nExit") -> ("States Out"=w419:string)  [unwired: 13 in]
        n149 = call <vilib>:"Add State(s) to Queue__jki_lib_state_machine.vi"("State(s) in Front (\"\")"=w419, "State(s) in (\"\")"=w423) -> ("States Out"=w422:string)  [unwired: 13 in]
      }
      frame "---------- Actions ----------" {
        n150 = call <vilib>:"Add State(s) to Queue__jki_lib_state_machine.vi"("State(s) in (\"\")"=w428) -> ("States Out"=w427:string)  [unwired: 14 in]
      }
      frame "Actions: Sort Volume" {
        n151 = Unbundle By Name(w436) -> ("current_vol_array"=w435:cluster{"name":string, "path":path}[], "root paths.cv_issues"=w434:path)
        n152 = local read "volumes"() -> (w431:i32)
        n153 = Index Array(array=w435, index=w431) -> (element=w430:cluster{"name":string, "path":path})
        n154 = Unbundle By Name(w430) -> ("path"=w429:path)
        n155 = call "sort.volume.issues.vi"("error in"=w437, "issues path"=w434, "volume path"=w429) -> ("error out"=w433:errorcluster)  [unwired: 8 in]
        n156 = property on="volumes" class="LstBox (strict)"(error in=w433, "Val(Sgnl)"=w431) -> (error out=w432:errorcluster)  [unwired: 1 in, 1 out]
        n157 = call <vilib>:"Add State(s) to Queue__jki_lib_state_machine.vi"("State(s) in (\"\")"=w440) -> ("States Out"=w439:string)  [unwired: 14 in]
      }
      frame "Actions: Move Issue Up" {
        n158 = Unbundle By Name(w459) -> ("current_vol_array"=w447:cluster{"name":string, "path":path}[], "volume"=w453:T3, "volume.issue_ids"=w458:i32[])
        n159 = local read "volumes"() -> (w444:i32)
        n160 = local read "issues"() -> (w454:i32)
        n161 = Index Array(array=w447, index=w444) -> (element=w446:cluster{"name":string, "path":path})
        n162 = Delete From Array(array=w458, length=1, index=w454) -> (deleted portion=w455:i32[], array with subset deleted=w456:i32[])
        n163 = Decrement(x=w454) -> (x-1=w441:i32)
        n164 = Unbundle By Name(w446) -> ("path"=w445:path)
        n165 = Insert Into Array(array=w456, index=w441, new element=w455) -> (w452:i32[])
        n166 = local write "issues"(w441) -> ()
        n167 = Bundle By Name(cluster=w453, "issue_ids"=w452) -> (w451:T3)
        n168 = call <vilib>:"Flatten To JSON String.vi"("error in (no error)"=w449, "Variant"=w451) -> ("error out"=w450:errorcluster, "JSON String"=w448:string)  [unwired: 8 in]
        n169 = Write to Text File(file (use dialog)=w445, text=w448, error in=w450) -> (error out=w443:errorcluster)  [unwired: 1 in, 2 out]
        n170 = property on="volumes" class="LstBox (strict)"(error in=w443, "Val(Sgnl)"=w444) -> (error out=w442:errorcluster)  [unwired: 1 in, 1 out]
        n171 = call <vilib>:"Add State(s) to Queue__jki_lib_state_machine.vi"("State(s) in (\"\")"=w462) -> ("States Out"=w461:string)  [unwired: 14 in]
      }
      frame "Actions: Move Issue Top" {
        w464 = 0 ("issues")
        n172 = Unbundle By Name(w483) -> ("current_vol_array"=w471:cluster{"name":string, "path":path}[], "volume"=w477:T3, "volume.issue_ids"=w482:i32[])
        n173 = local read "volumes"() -> (w468:i32)
        n174 = local read "issues"() -> (w478:i32)
        n175 = Index Array(array=w471, index=w468) -> (element=w470:cluster{"name":string, "path":path})
        n176 = Delete From Array(array=w482, length=1, index=w478) -> (deleted portion=w479:i32[], array with subset deleted=w480:i32[])
        n177 = Unbundle By Name(w470) -> ("path"=w469:path)
        n178 = Insert Into Array(array=w480, index=0, new element=w479) -> (w476:i32[])
        n179 = Bundle By Name(cluster=w477, "issue_ids"=w476) -> (w475:T3)
        n180 = call <vilib>:"Flatten To JSON String.vi"("error in (no error)"=w473, "Variant"=w475) -> ("error out"=w474:errorcluster, "JSON String"=w472:string)  [unwired: 8 in]
        n181 = Write to Text File(file (use dialog)=w469, text=w472, error in=w474) -> (error out=w467:errorcluster)  [unwired: 1 in, 2 out]
        n182 = property on="volumes" class="LstBox (strict)"(error in=w467, "Val(Sgnl)"=w468) -> (error out=w466:errorcluster)  [unwired: 1 in, 1 out]
        n183 = property on="issues" class="LstBox (strict)"(error in=w466, "Value"=w464, "Top Row"=w464) -> (error out=w465:errorcluster)  [unwired: 1 in, 1 out]
        n184 = call <vilib>:"Add State(s) to Queue__jki_lib_state_machine.vi"("State(s) in (\"\")"=w486) -> ("States Out"=w485:string)  [unwired: 14 in]
      }
      frame "Actions: Move Issue Down" {
        n185 = Unbundle By Name(w505) -> ("current_vol_array"=w493:cluster{"name":string, "path":path}[], "volume"=w499:T3, "volume.issue_ids"=w504:i32[])
        n186 = local read "volumes"() -> (w490:i32)
        n187 = local read "issues"() -> (w500:i32)
        n188 = Index Array(array=w493, index=w490) -> (element=w492:cluster{"name":string, "path":path})
        n189 = Delete From Array(array=w504, length=1, index=w500) -> (deleted portion=w501:i32[], array with subset deleted=w502:i32[])
        n190 = Increment(x=w500) -> (x+1=w487:i32)
        n191 = Unbundle By Name(w492) -> ("path"=w491:path)
        n192 = Insert Into Array(array=w502, index=w487, new element=w501) -> (w498:i32[])
        n193 = local write "issues"(w487) -> ()
        n194 = Bundle By Name(cluster=w499, "issue_ids"=w498) -> (w497:T3)
        n195 = call <vilib>:"Flatten To JSON String.vi"("error in (no error)"=w495, "Variant"=w497) -> ("error out"=w496:errorcluster, "JSON String"=w494:string)  [unwired: 8 in]
        n196 = Write to Text File(file (use dialog)=w491, text=w494, error in=w496) -> (error out=w489:errorcluster)  [unwired: 1 in, 2 out]
        n197 = property on="volumes" class="LstBox (strict)"(error in=w489, "Val(Sgnl)"=w490) -> (error out=w488:errorcluster)  [unwired: 1 in, 1 out]
        n198 = call <vilib>:"Add State(s) to Queue__jki_lib_state_machine.vi"("State(s) in (\"\")"=w508) -> ("States Out"=w507:string)  [unwired: 14 in]
      }
      frame "Actions: Load Volume" {
        w514 = T3 {"id"=0, "name"="", "name_sortable"="", "aliases"=[], "description"="", "url"="", "count_of_issues"=0, "start_year"=0, "publisher_id"=0, "issue_ids"=[], "date_last_updated"=timestamp(0 s since 1904-01-01), "volume"=0, "cv_id"=""} ("volume")
        n199 = Unbundle By Name(w511) -> ("current_vol_array"=w523:cluster{"name":string, "path":path}[])
        n200 = local read "volumes"() -> (w522:i32)
        n201 = Index Array(array=w523, index=w522) -> (element=w521:cluster{"name":string, "path":path})
        n202 = Unbundle By Name(w521) -> ("path"=w520:path)
        n203 = Read from Text File(file (use dialog)=w520, error in=w519) -> (text=w517:string, error out=w518:errorcluster)  [unwired: 2 in, 2 out]
        n204 = call <vilib>:"Unflatten From JSON String.vi"("Type and Defaults"=w514, "error in (no error)"=w518, "JSON String"=w517) -> ("error out"=w516:errorcluster, "Variant"=w515:variant)  [unwired: 7 in]
        n205 = Variant To Data(error in=w516, type=w514, Variant=w515) -> (data=w509:T3, error out=w513:errorcluster)
        n206 = Bundle By Name(cluster=w511, "volume"=w509) -> (w510:T8)
        n207 = call <vilib>:"Add State(s) to Queue__jki_lib_state_machine.vi"("State(s) in (\"\")"=w525) -> ("States Out"=w524:string)  [unwired: 14 in]
      }
      frame "Actions: Load Issues" {
        n208 = Unbundle By Name(w530) -> ("root paths.cv_issues"=w526:path, "volume.issue_ids"=w533:i32[])
        n209 = for {
          tunnel: w533 -> [w547] mode=indexing
          tunnel: "%d.json" -> [w548]
          tunnel: w526 -> [w545]
          shift-right: [w539] -> w527
          shift-left: w531 -> [w543]
          tunnel: [w538] -> w529 mode=indexing if=w537
          n210 = Format Into String(format string=w548, w547) -> (resulting string=w546:string)  [unwired: 2 in, 1 out]
          n211 = Build Path(base path=w545, name or relative path=w546) -> (appended path=w544:path)
          n212 = call <vilib>:"Check if File or Folder Exists.vi"("error in (no error)"=w543, "path"=w544) -> ("error out"=w540:errorcluster, "file or folder exists?"=w542:bool, "dup path"=w541:path)  [unwired: 7 in]
          n213 = case shown="False" w542 {
            selector: w542 -> [w549 w551]
            tunnel: w541 -> [_ w560]
            tunnel: w540 -> [w550 w559]
            tunnel: [_ w553] -> w538
            tunnel: [w550 w552] -> w539
            tunnel: [w549 w551] -> w537
            frame False {
            }
            frame True {
              w554 = T4 {"cover_date"=timestamp(0 s since 1904-01-01), "id"=0, "cv_id"="", "name"="", "sortable_name"="", "issue_number"="", "deck"="", "description"="", "volume"={"id"=0, "name"=""}, "store_date"=timestamp(0 s since 1904-01-01), "date_last_updated"=timestamp(0 s since 1904-01-01), "site_detail_url"="", "cover_url"="", "associated_images"=[], "characters"=[], "concepts"=[], "creators"=[], "storyArcs"=[], "teams"=[]} ("issue")
              n214 = Read from Text File(file (use dialog)=w560, error in=w559) -> (text=w557:string, error out=w558:errorcluster)  [unwired: 2 in, 2 out]
              n215 = call <vilib>:"Unflatten From JSON String.vi"("Type and Defaults"=w554, "error in (no error)"=w558, "JSON String"=w557) -> ("error out"=w556:errorcluster, "Variant"=w555:variant)  [unwired: 7 in]
              n216 = Variant To Data(error in=w556, type=w554, Variant=w555) -> (data=w553:T4, error out=w552:errorcluster)
            }
          }
        }
        n217 = Bundle By Name(cluster=w530, "issues"=w529) -> (w528:T8)
        n218 = call <vilib>:"Add State(s) to Queue__jki_lib_state_machine.vi"("State(s) in (\"\")"=w536) -> ("States Out"=w535:string)  [unwired: 14 in]
      }
      frame "Actions: Populate cv_vols" {
        n219 = Unbundle By Name(w562) -> ("root paths.cv_volumes"=w561:path)
        n220 = call <vilib>:"Recursive File List.vi"("pattern"="*.json", "error in (no error)"=w564, "Folder Path"=w561) -> ("error out"=w565:errorcluster, "All Files in Dir"=w567:path[])  [unwired: 4 in, 3 out]
        n221 = Bundle By Name(cluster=w562, "cv_vols"=w567) -> (w566:T8)
        n222 = call <vilib>:"Add State(s) to Queue__jki_lib_state_machine.vi"("State(s) in (\"\")"=w570) -> ("States Out"=w569:string)  [unwired: 14 in]
      }
      frame "Actions: create volume filter map" {
        n223 = property on="Folder" class="LstBox (strict)"(error in=w572) -> (error out=w573:errorcluster, "Item Names"=w580:string[])  [unwired: 1 in, 1 out]
        n224 = Unbundle By Name(w576) -> ("cv_vols"=w578:path[])
        n225 = To Lower Case(string=w580) -> (all lower case string=w579:string[])
        n226 = for {
          tunnel: w579 -> [w591]
          tunnel: w578 -> [w590] mode=indexing
          shift-right: [w585] -> w575
          shift-left: map{i32, cluster{"name":string, "path":path}[]} {} ("map") -> [w587]
          n227 = Strip Path(path=w590) -> (name=w594:string)  [unwired: 1 out]
          n228 = call-poly <userlib>:"Strip Path Extension__ogtk.vi"("path"=w594) -> ("root"=w582:string)  [unwired: 1 out]
          n229 = String Subset(string=w582, length (rest)=1 ("length (rest)")) -> (substring=w592:string)  [unwired: 1 in]
          n230 = Decimal String To Number(string=w592) -> (offset past number=w593:i32)  [unwired: 2 in, 1 out]
          n231 = case shown="0" w593 {
            tunnel: w592 -> [w607 _]
            tunnel: w591 -> [w608 _]
            tunnel: [w606 0 ("index of element")] -> w586
            frame 0 {
              n232 = Search 1D Array(1D array=w608, element=w607) -> (index of element=w606:i32)  [unwired: 1 in]
            }
            frame Default {
            }
          }
          n233 = Bundle("root"=w582, "cv_vols"=w590) -> (w589:cluster{"root":string, "cv_vols":path})  [unwired: 1 in]
          n234 = Look In Map(map=w587, key=w586) -> (key not found?=w588:bool, value=w584:cluster{"name":string, "path":path}[])  [unwired: 1 in]
          n235 = case shown="True" w588 {
            tunnel: w589 -> [w598 w603]
            tunnel: w587 -> [w597 w605]
            tunnel: w586 -> [w595 w604]
            tunnel: [w596 w601] -> w585
            tunnel: w584 -> [w599 _]
            frame False {
              n236 = Build Array (concatenate)(w599, w598) -> (w600:cluster{"root":string, "cv_vols":path}[])
              n237 = Insert Into Map(map in=w597, key=w595, value=w600) -> (map out=w596:map{i32, cluster{"name":string, "path":path}[]})  [unwired: 2 out]
            }
            frame True {
              n238 = Build Array(w603) -> (w602:cluster{"root":string, "cv_vols":path}[])
              n239 = Insert Into Map(map in=w605, key=w604, value=w602) -> (map out=w601:map{i32, cluster{"name":string, "path":path}[]})  [unwired: 2 out]
            }
          }
        }
        n240 = Bundle By Name(cluster=w576, "vol_filter_map"=w575) -> (w574:T8)
      }
    }
  }
